vi "Array with 4 elements.vi"(10 "Array with 4 elements":dbl[](array[numeric])) -> (0 "element 3":dbl, 1 "element 2":dbl, 2 "element 1":dbl, 3 "element 0":dbl)   [LabVIEW 2016]
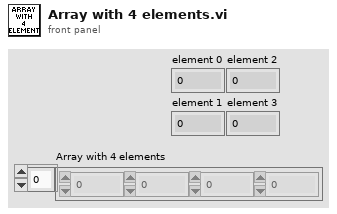
[diagram p1: front panel]
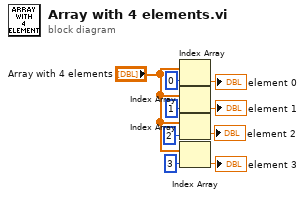
[diagram p0: block diagram]
diagram:
  n1 = Index Array(array="Array with 4 elements", index=0) -> (element=→"element 0":dbl)
  n2 = Index Array(array="Array with 4 elements", index=1) -> (element=→"element 1":dbl)
  n3 = Index Array(array="Array with 4 elements", index=2) -> (element=→"element 2":dbl)
  n4 = Index Array(array="Array with 4 elements", index=3) -> (element=→"element 3":dbl)
